vi "OCU_Main.vi"() -> ()   [LabVIEW 2013]
doc: "To be executed on the Opperator Control Unit (laptop), which communicates to a variety of platforms for the sailbot boat to send missions to complete, override commands, and to monitor the status of the boat and parts of the code run on it. It should be run in parallel with \"Main.vi\" in the cRIO code foler. \n\nCreaded by Victoria Coleman and Elizabeth Mahon (03/14)"
uses:
  cRIO_Code/Data/TypeDefs/MissionTypeControl.ctl
  cRIO_Code/Data/TypeDefs/UTM Location.ctl
  cRIO_Code/Data/TypeDefs/MissionDescription.ctl
  cRIO_Code/Data/TypeDefs/MainsailPositionIndicator.ctl
  cRIO_Code/Data/TypeDefs/JibPositionIndicator.ctl
  cRIO_Code/Data/TypeDefs/Rudder Set Suggestions.ctl
  cRIO_Code/Data/TypeDefs/OverrideMode.ctl
  cRIO_Code/Data/TypeDefs/MotorSetup.ctl
  cRIO_Code/Data/TypeDefs/DynamixelSetupInfo.ctl
  cRIO_Code/Logic/Classes/Missions/GenericMission/GenericMission.lvclass
  Location of Think.ctl
  RIO-OCU_Comm/ToRIO.ctl
  CommandMessages.ctl
  cRIO_Code/Logic/Classes/Missions/GoTo/GoTo.lvclass
  cRIO_Code/Logic/Classes/Missions/RoundBouy/RoundBouy.lvclass
  cRIO_Code/Logic/Classes/Missions/PassBouy/PassBouy.lvclass
  cRIO_Code/Logic/Classes/Missions/StationKeeping/StationKeeping.lvclass
  RIO-OCU_Comm/NetworkStreams/Writer/NetworkStreamWriter.lvclass
panel:
  in  "Cluster":T1
  in  "OverrideMode":T3
  in  "Boat Type":T4(ring)=enum."Simulation"
  in  "Tab Control":enum32{"Mission Management", "Manual Control"}(tab)
  in  "CreateMission":bool
  in  "Mission Type":T5
  in  "Points of Interest":T6[](array[typedef]) {"North" format="%#_10f"; "East" format="%#_8f"}
  in  "Tolerance (m)":dbl
  in  "Duration (s)":dbl=-1.0
  in  "Timeout (s)":dbl=-1.0
  out "# of Missions":i32
  in  "ID# To Delete":u16
  in  "DeleteMission":bool
  out "Current Missions":T7[](array[typedef]) {"Points of Interest"."North" format="%#_10f"; "Points of Interest"."East" format="%#_8f"}
  in  "Mainsail Position":T8
  in  "Jib Position":T9
  in  "Rudder Setpoint":T10 min=-1.0 max=1.0 scale=1.0..-1.0
  out "error out":errorcluster
  out "Connected?":bool
  in  "stop":bool
  # "RUN MAIN.VI FIRST. SERIOUSLY"
  # "If you forgot to set the boat type, you must restart the code"
  # "TODO: Add in the clickable map"
  # "TODO: When you delete the last mission, make idle take its place. Then when the next mission is initialized, delete the idle mission"
  # "KEY MAPPINGS TO ACTUATOR MOVEMENT:\n\"Page Up\" -- rudder right       |    \"Up\" -- Main out          |     \"Page Down\" -- Jib out\n\"Left\" -- rudder left                  |      \"Down\" -- Main in     |      \"Right\" -- Jib in"
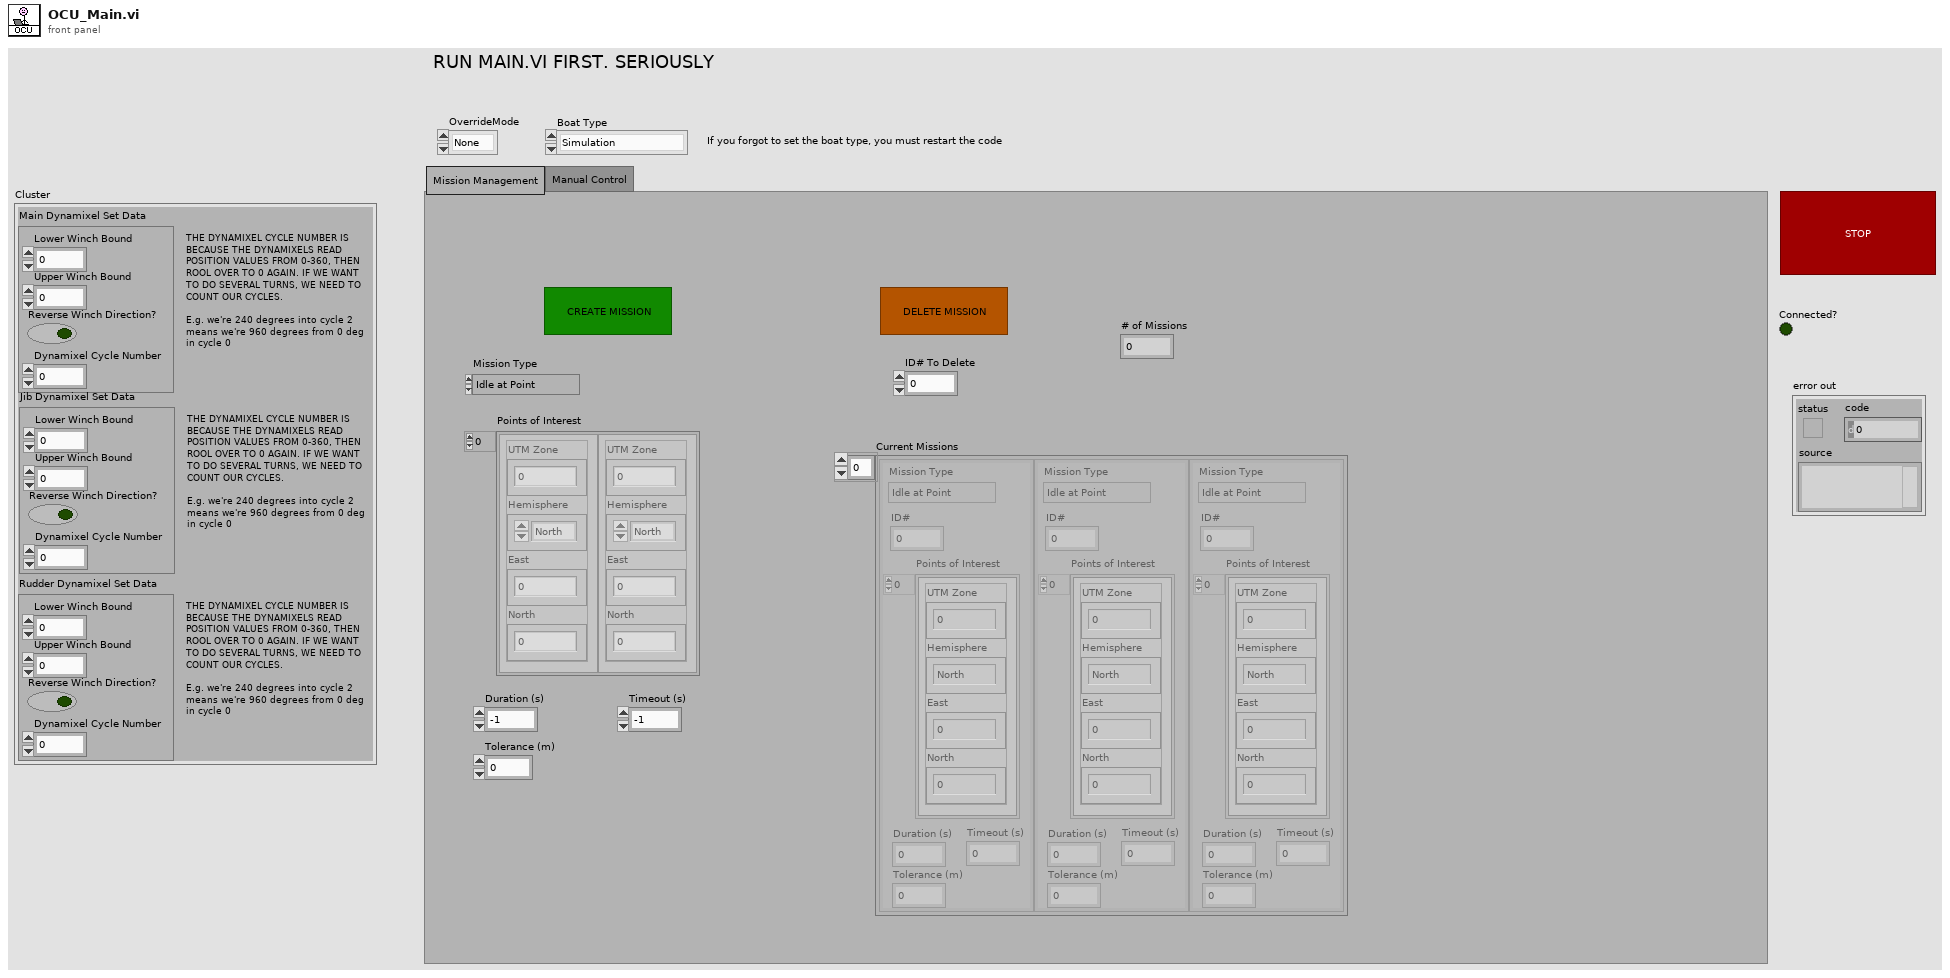
[diagram p1: front panel]
types:
  T1 = typedef "MotorSetup.ctl" = cluster{"Main Dynamixel Set Data":T2, "Rudder Dynamixel Set Data":T2, "Jib Dynamixel Set Data":T2}
  T2 = typedef "DynamixelSetupInfo.ctl" = cluster{"Lower Winch Bound":dbl, "Upper Winch Bound":dbl, "Reverse Winch Direction?":bool, "Dynamixel Cycle Number":i32}
  T3 = typedef "OverrideMode.ctl" = enum16{"None", "Rudder", "Sails", "Both"}
  T4 = enum16{"Blackbody Radiation", "Little boats", "Simulation", "Damn Yankee"}
  T5 = typedef "MissionTypeControl.ctl" = enum16{"Idle at Point", "Drive to Waypoint", "Round Buoy to Port", "Round Buoy to Starboard", "Pass Between Buoys", "Station Keeping"}
  T6 = typedef "UTM Location.ctl" = cluster{"UTM Zone":dbl, "Hemisphere":enum16{"North", "South"}, "East":dbl, "North":dbl}
  T7 = typedef "MissionDescription.ctl" = cluster{"Duration (s)":dbl, "Timeout (s)":dbl, "Tolerance (m)":dbl, "Mission Type":T5, "Points of Interest":T6[], "ID#":i32}
  T8 = typedef "MainsailPositionIndicator.ctl" = dbl
  T9 = typedef "JibPositionIndicator.ctl" = dbl
  T10 = typedef "Rudder Set Suggestions.ctl" = dbl
  T11 = typedef "CommandMessages.ctl" = enum16{"Boat Type", "Pass", "OverrideMode", "Add mission", "Delete mission", "Change constants"}
  T12 = typedef "ToRIO.ctl" = cluster{"Commands":T11, "Variant":variant}
  T13 = typedef "Location of Think.ctl" = string
  T14 = typedef "eventvkey.ctl" = enum16{"ASCII", "Enter", "Return", "Shift", "Ctrl", "Alt", "Cmd", "Opt", "Caps", "NumLock", "Clear", "Break", "Up", "Down", "Left", "Right", "Insert", "Delete", "Home", "End", "PageUp", "PageDown", "Escape", "Help", "Pause", "ScrollLock", "F1", "F2", "F3", "F4", "F5", "F6", "F7", "F8", "F9", "F10", "F11", "F12", "F13", "F14", "F15", "F16", "F17", "F18", "F19", "F20", "F21", "F22", "F23", "F24", "Play", "VolumeUp", "VolumeDown", "Mute", "Two Byte Char"}
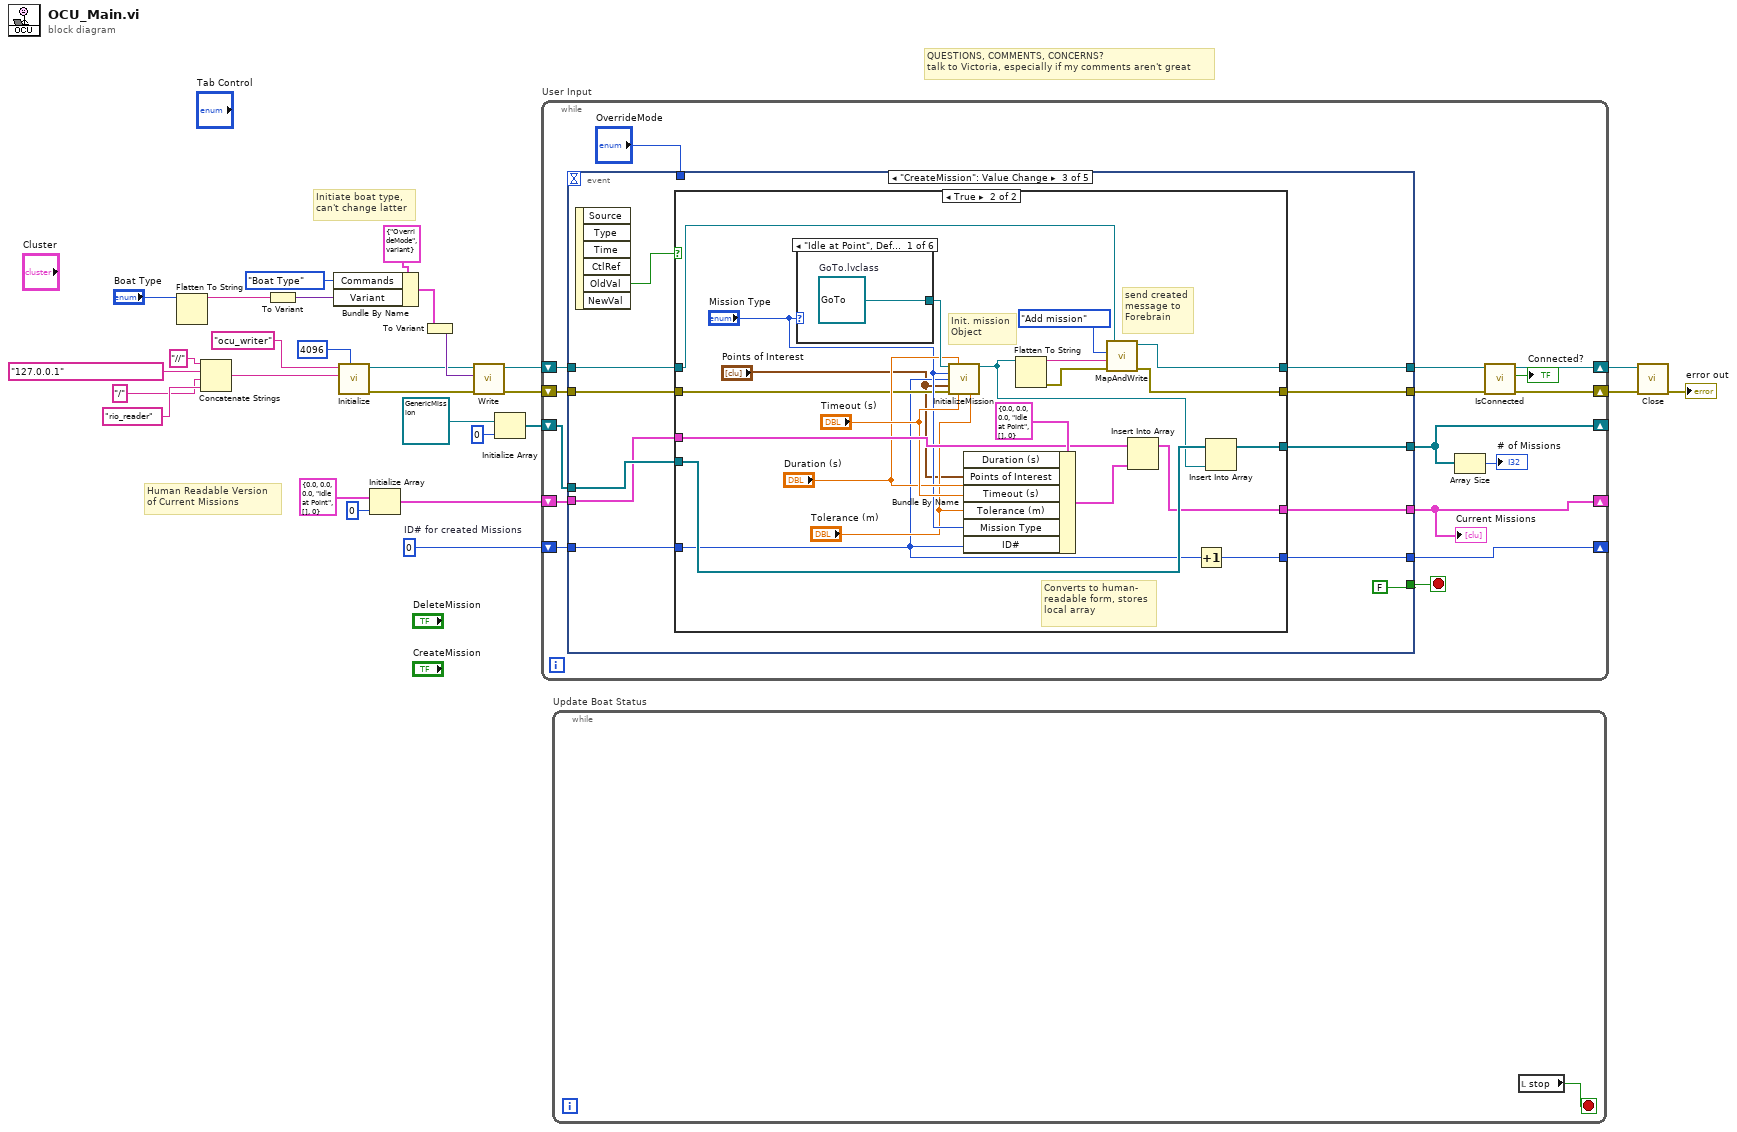
[diagram p0: block diagram]
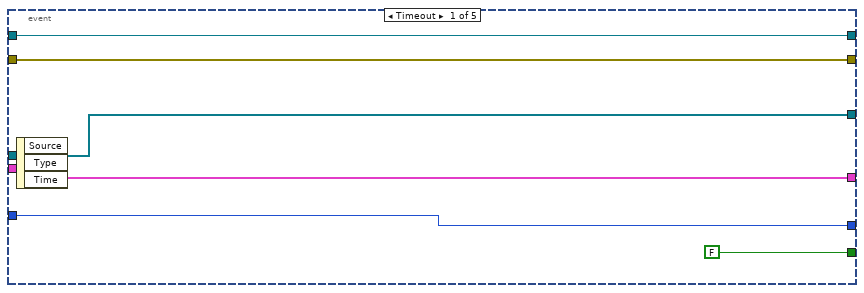
[diagram p2: hidden frame]
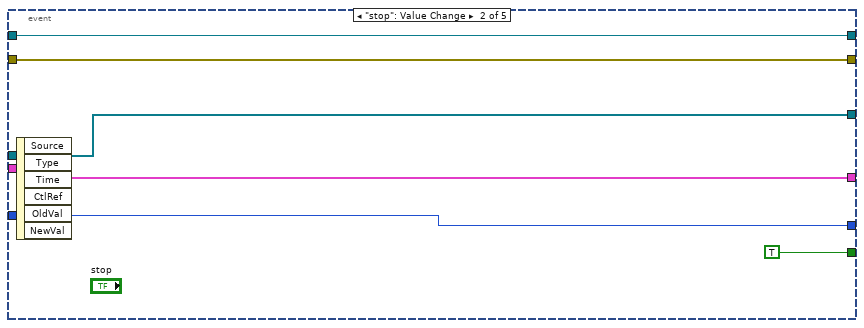
[diagram p3: hidden frame]
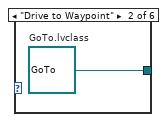
[diagram p5: hidden frame]
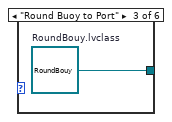
[diagram p6: hidden frame]
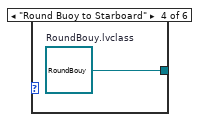
[diagram p7: hidden frame]
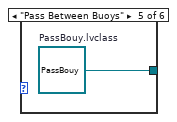
[diagram p8: hidden frame]
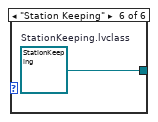
[diagram p9: hidden frame]
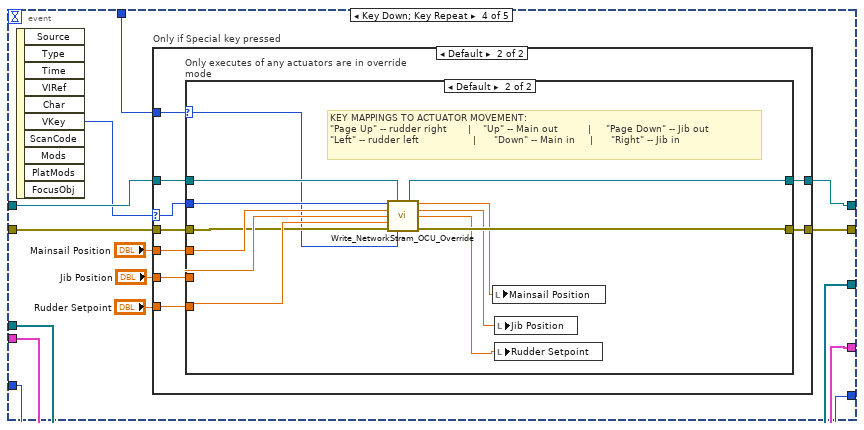
[diagram p10: hidden frame]
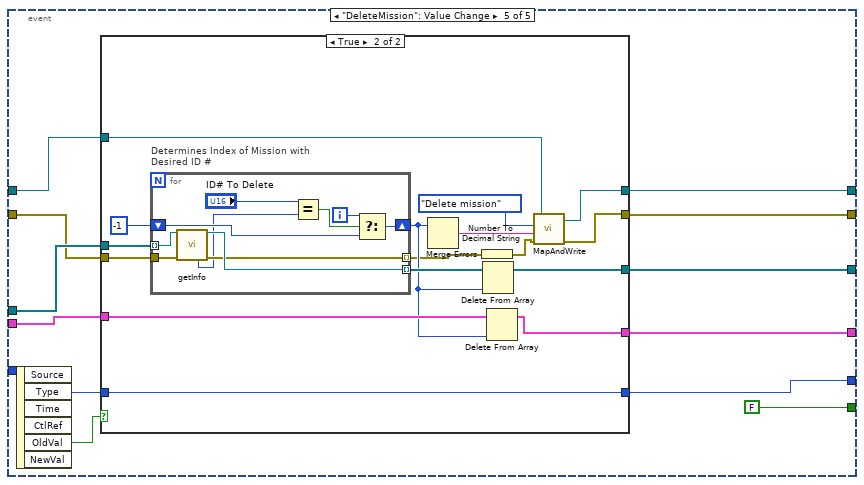
[diagram p13: hidden frame]
diagram:
  w6 = 0  # ID# for created Missions
  # "Initiate boat type,\ncan't change latter"
  # "QUESTIONS, COMMENTS, CONCERNS? \ntalk to Victoria, especially if my comments aren't great"
  # "Human Readable Version\nof Current Missions"
  n1 = Flatten To String(anything="Boat Type") -> (data string=w1:string)  [unwired: 3 in, 2 out]
  n2 = Concatenate Strings("//" ("string"), T13 "127.0.0.1" ("Location of THINK"), "/", "rio_reader" ("string")) -> (w19:string)
  n3 = To Variant(anything=w1) -> (Variant=w4:variant)
  n4 = Bundle By Name(cluster=T12 {"Commands"=enum."OverrideMode", "Variant"=variant} ("To RIO"), "Commands"=CommandMessages."Boat Type", "Variant"=w4) -> (w3:T12)
  n5 = call "Initialize.vi"("writer buffer size"=4096, "reader url"=w19, "writer name"="ocu_writer") -> ("error out"=w9:errorcluster, "NetworkStreamWriter out"=w10:refnum<class "NetworkStreamWriter.lvclass">)  [unwired: 7 in]
  n6 = Initialize Array(T7 {"Duration (s)"=0.0, "Timeout (s)"=0.0, "Tolerance (m)"=0.0, "Mission Type"=enum."Idle at Point", "Points of Interest"=[], "ID#"=0} ("input cluster"), 0 ("dimension size")) -> (w24:T7[])
  n7 = To Variant(anything=w3) -> (Variant=w12:variant)
  n8 = call "Write.vi"("error in (no error)"=w9, "element"=w12, "NetworkStreamWriter in"=w10) -> ("error out"=w8:errorcluster, "NetworkStreamWriter out"=w7:refnum<class "NetworkStreamWriter.lvclass">)  [unwired: 7 in]
  n9 = Initialize Array(refnum<class "GenericMission.lvclass"> refnum ("GenericMission.lvclass"), 0 ("dimension size")) -> (w27:refnum<class "GenericMission.lvclass">[])
  n10 = while "User Input" {
    shift-right: [w38] -> _
    shift-left: w27 -> [w44]
    shift-right: [w42] -> _
    shift-left: w6 -> [w43]
    shift-right: [w39] -> _
    shift-left: w24 -> [w40]
    shift-right: [w31] -> w17
    shift-left: w8 -> [w36]
    shift-right: [w33] -> w18
    shift-left: w7 -> [w35]
    stop <- w37 stop-if-true
    n11 = event shown="[2] \"CreateMission\": Value Change" {
      selector: _ -> [_ _ _ _ _]
      dyn-events: _ -> [_ _ _ _ _]
      timeout: _ -> [_ _ _ _ _]
      tunnel: w44 -> [w49 w55 w67 w110 w150]
      tunnel: [w49 w55 w66 w110 w149] -> w38
      tunnel: w43 -> [w50 w54 w68 w112 w144]
      tunnel: [w50 w54 w62 w112 w145] -> w42
      tunnel: w40 -> [w47 w53 w65 w111 w148]
      tunnel: [w47 w53 w64 w111 w147] -> w39
      tunnel: [FALSE TRUE FALSE _ FALSE] -> w37
      tunnel: [w46 w52 w60 w107 w142] -> w32
      tunnel: w35 -> [w45 w51 w59 w113 w140]
      tunnel: w36 -> [w46 w52 w58 w108 w141]
      tunnel: [w45 w51 w57 w109 w139] -> w34
      tunnel: "OverrideMode" -> [_ _ _ w102 _]
      event Timeout {
        n12 = event-data() -> ()  [unwired: 1 in, 3 out]
      }
      event "stop": Value Change {
        n13 = event-data() -> ()  [unwired: 1 in, 6 out]
      }
      event "CreateMission": Value Change {
        n14 = event-data() -> ("OldVal"=w61:bool)  [unwired: 1 in, 5 out]
        n15 = case shown="True" w61 {
          tunnel: w68 -> [w71 w81]
          tunnel: w67 -> [w73 w94]
          tunnel: [w73 w93] -> w66
          tunnel: w65 -> [w72 w90]
          tunnel: [w72 w89] -> w64
          tunnel: [w71 w84] -> w62
          tunnel: [w70 w74] -> w60
          tunnel: w59 -> [w69 w78]
          tunnel: w58 -> [w70 w83]
          tunnel: [w69 w75] -> w57
          frame False {
          }
          frame True {
            # "Init. mission\nObject"
            # "send created\nmessage to\nForebrain"
            # "Converts to human-\nreadable form, stores\nlocal array"
            n16 = case shown="\"Idle at Point\", Default" "Mission Type" {
              tunnel: [w96 w97 w98 w99 w100 w101] -> w95
              frame "Idle at Point", Default {
                w96 = refnum<class "GoTo.lvclass"> refnum  # GoTo.lvclass
              }
              frame "Drive to Waypoint" {
                w97 = refnum<class "GoTo.lvclass"> refnum  # GoTo.lvclass
              }
              frame "Round Buoy to Port" {
                w98 = refnum<class "RoundBouy.lvclass"> refnum  # RoundBouy.lvclass
              }
              frame "Round Buoy to Starboard" {
                w99 = refnum<class "RoundBouy.lvclass"> refnum  # RoundBouy.lvclass
              }
              frame "Pass Between Buoys" {
                w100 = refnum<class "PassBouy.lvclass"> refnum  # PassBouy.lvclass
              }
              frame "Station Keeping" {
                w101 = refnum<class "StationKeeping.lvclass"> refnum  # StationKeeping.lvclass
              }
            }
            n17 = call-dynamic "InitializeMission.vi"("GenericMission in"=w95, "Duration (s)"="Duration (s)", "Mission Type"="Mission Type", "ID#"=w81, "Points of Interest"="Points of Interest", "Error In"=w83, "Timeout (s)"="Timeout (s)", "Tolerance (m)"="Tolerance (m)") -> ("GenericMission out"=w82:refnum<class "GenericMission.lvclass">)  [unwired: 6 in, 1 out]
            n18 = Bundle By Name(cluster=T7 {"Duration (s)"=0.0, "Timeout (s)"=0.0, "Tolerance (m)"=0.0, "Mission Type"=enum."Idle at Point", "Points of Interest"=[], "ID#"=0} ("input cluster"), "Duration (s)"="Duration (s)", "Points of Interest"="Points of Interest", "Timeout (s)"="Timeout (s)", "Tolerance (m)"="Tolerance (m)", "Mission Type"="Mission Type", "ID#"=w81) -> (w91:T7)
            n19 = Flatten To String(anything=w82) -> (data string=w77:string, error out=w76:errorcluster)  [unwired: 3 in, 1 out]
            n20 = call "MapAndWrite.vi"("error in (no error)"=w76, "String_Cast_of_Info"=w77, "Commands"=CommandMessages."Add mission", "NetworkStreamWriter in"=w78) -> ("error out"=w74:errorcluster, "NetworkStreamWriter out"=w75:refnum<class "NetworkStreamWriter.lvclass">)  [unwired: 2 in]
            n21 = Insert Into Array(array=w90, new element=w91) -> (w89:T7[])  [unwired: 1 in]
            n22 = Increment(x=w81) -> (x+1=w84:i32)
            n23 = Insert Into Array(array=w94, new element=w82) -> (w93:refnum<class "GenericMission.lvclass">[])  [unwired: 1 in]
          }
        }
      }
      event Key Down; Key Repeat {
        n24 = event-data() -> ("VKey"=w103:T14)  [unwired: 1 in, 9 out]
        n25 = case "Only if Special key pressed" shown="Default" w103 {
          selector: w103 -> [_ w121]
          tunnel: w113 -> [w115 w117]
          tunnel: [w115 w118] -> w109
          tunnel: w108 -> [w114 w120]
          tunnel: [w114 w119] -> w107
          tunnel: "Rudder Setpoint" -> [_ w124]
          tunnel: "Jib Position" -> [_ w123]
          tunnel: "Mainsail Position" -> [_ w122]
          tunnel: w102 -> [_ w116]
          frame "ASCII" {
            # "No special key pressed :("
          }
          frame Default {
            n26 = case "Only executes of any actuators are in override mode" shown="Default" w116 {
              selector: w116 -> [_ w131]
              tunnel: w124 -> [_ w136]
              tunnel: w123 -> [_ w137]
              tunnel: w122 -> [_ w138]
              tunnel: w121 -> [_ w134]
              tunnel: w120 -> [w126 w133]
              tunnel: [w126 w135] -> w119
              tunnel: [w125 w130] -> w118
              tunnel: w117 -> [w125 w132]
              frame "None" {
              }
              frame Default {
                # "KEY MAPPINGS TO ACTUATOR MOVEMENT:\n\"Page Up\" -- rudder right       |    \"Up\" -- Main out          |     \"Page Down\" -- Jib out\n\"Left\" -- rudder left                  |      \"Down\" -- Main in     |      \"Right\" -- Jib in"
                n27 = call "Write_NetworkStram_OCU_Override.vi"("VKey"=w134, "NetworkStreamWriter in"=w132, "Mainsail Position"=w138, "Jib Position"=w137, "Rudder Setpoint"=w136, "error in (no error)"=w133, "OverrideMode"=w131) -> ("NetworkStreamWriter out"=w130:refnum<class "NetworkStreamWriter.lvclass">, "Main Position"=w129:T8, "Jib Position"=w128:T9, "Rudder Position"=w127:T10, "error out"=w135:errorcluster)  [unwired: 4 in]
                n28 = local write "Mainsail Position"(w129) -> ()
                n29 = local write "Jib Position"(w128) -> ()
                n30 = local write "Rudder Setpoint"(w127) -> ()
              }
            }
          }
        }
      }
      event "DeleteMission": Value Change {
        n31 = event-data() -> ("OldVal"=w143:bool)  [unwired: 1 in, 5 out]
        n32 = case shown="True" w143 {
          tunnel: w150 -> [w155 w171]
          tunnel: [w155 w159] -> w149
          tunnel: w148 -> [w154 w168]
          tunnel: [w154 w167] -> w147
          tunnel: [w153 w166] -> w145
          tunnel: w144 -> [w153 w166]
          tunnel: [w152 w157] -> w142
          tunnel: w141 -> [w152 w164]
          tunnel: w140 -> [w151 w163]
          tunnel: [w151 w156] -> w139
          frame False {
          }
          frame True {
            n33 = for "Determines Index of Mission with\nDesired ID #" {
              tunnel: w171 -> [w181] mode=indexing
              tunnel: [w180] -> w169 mode=indexing
              shift-right: [w177] -> w165
              shift-left: -1 -> [w176]
              tunnel: [w175] -> w160 mode=indexing
              tunnel: w164 -> [w174]
              i -> [w178]
              n34 = call-dynamic "getInfo.vi"("GenericMission in"=w181, "error in (no error)"=w174) -> ("GenericMission out"=w180:refnum<class "GenericMission.lvclass">, "ID#"=w172:u16, "error out"=w175:errorcluster)  [unwired: 5 in, 6 out]
              n35 = Equal?(x="ID# To Delete", y=w172) -> (x = y?=w179:bool)
              n36 = Select(t=w178, s=w179, f=w176) -> (s? t:f=w177:i32)
            }
            n37 = Number To Decimal String(number=w165) -> (decimal integer string=w161:string)  [unwired: 1 in]
            n38 = Merge Errors(w160) -> (w158:errorcluster)
            n39 = Delete From Array(array=w169, index=w165) -> (array with subset deleted=w159:refnum<class "GenericMission.lvclass">[])  [unwired: 1 in, 1 out]
            n40 = Delete From Array(array=w168, index=w165) -> (array with subset deleted=w167:T7[])  [unwired: 1 in, 1 out]
            n41 = call "MapAndWrite.vi"("error in (no error)"=w158, "String_Cast_of_Info"=w161, "Commands"=CommandMessages."Delete mission", "NetworkStreamWriter in"=w163) -> ("error out"=w157:errorcluster, "NetworkStreamWriter out"=w156:refnum<class "NetworkStreamWriter.lvclass">)  [unwired: 2 in]
          }
        }
      }
    }
    "Current Missions" <- w39
    n42 = Array Size(array=w38) -> (size(s)=→"# of Missions":i32)
    n43 = call "IsConnected.vi"("error in (no error)"=w32, "NetworkStreamWriter in"=w34) -> ("error out"=w31:errorcluster, "Connected?"=→"Connected?":bool, "NetworkStreamWriter out"=w33:refnum<class "NetworkStreamWriter.lvclass">)  [unwired: 7 in]
  }
  n44 = while "Update Boat Status" {
    stop <- w182 stop-if-true
    n45 = local read "stop"() -> (w182:bool)
  }
  n46 = call "Close.vi"("error in (no error)"=w17, "NetworkStreamWriter in"=w18) -> ("error out"=→"error out":errorcluster)  [unwired: 9 in]
